vi "P1.vi"() -> ()   [LabVIEW 2021]
panel:
  out "Boolean":bool
  in  "SP (PSI)":dbl
  out "PRESIÓN (PSI)":dbl(knob) scale=0.0..10.0
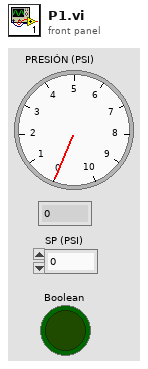
[diagram p1: front panel]
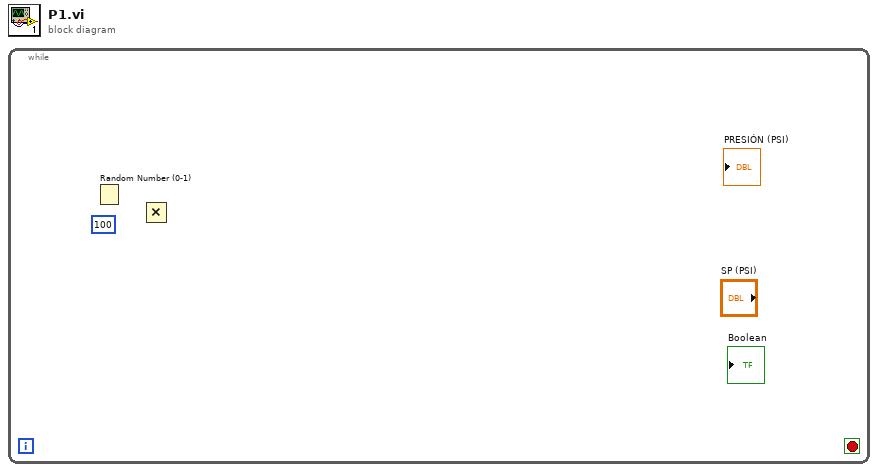
[diagram p0: block diagram]
diagram:
  n1 = while {
    stop <- _ stop-if-true
    (unwired) 100
    n2 = Random Number (0-1)() -> ()  [unwired: 1 out]
    n3 = Multiply() -> ()  [unwired: 2 in, 1 out]
  }
